vi "Sort_radius.vi"(2 "error in":errorcluster, 3 "unsorted array":dbl[][](array[numeric])) -> (0 "error out":errorcluster, 1 "Array":dbl[][](array[numeric]))   [LabVIEW 2016]
doc: "To vi sortuje tablice 1d pkt w tablice 2d pkt względem promienia , gdzie każdy wiersz to pkt z tym samym promieniem"
uses:
  <vilib>/express/express arith-compare/Formula/XNode/ExpressFormulaBlockNode.xnode
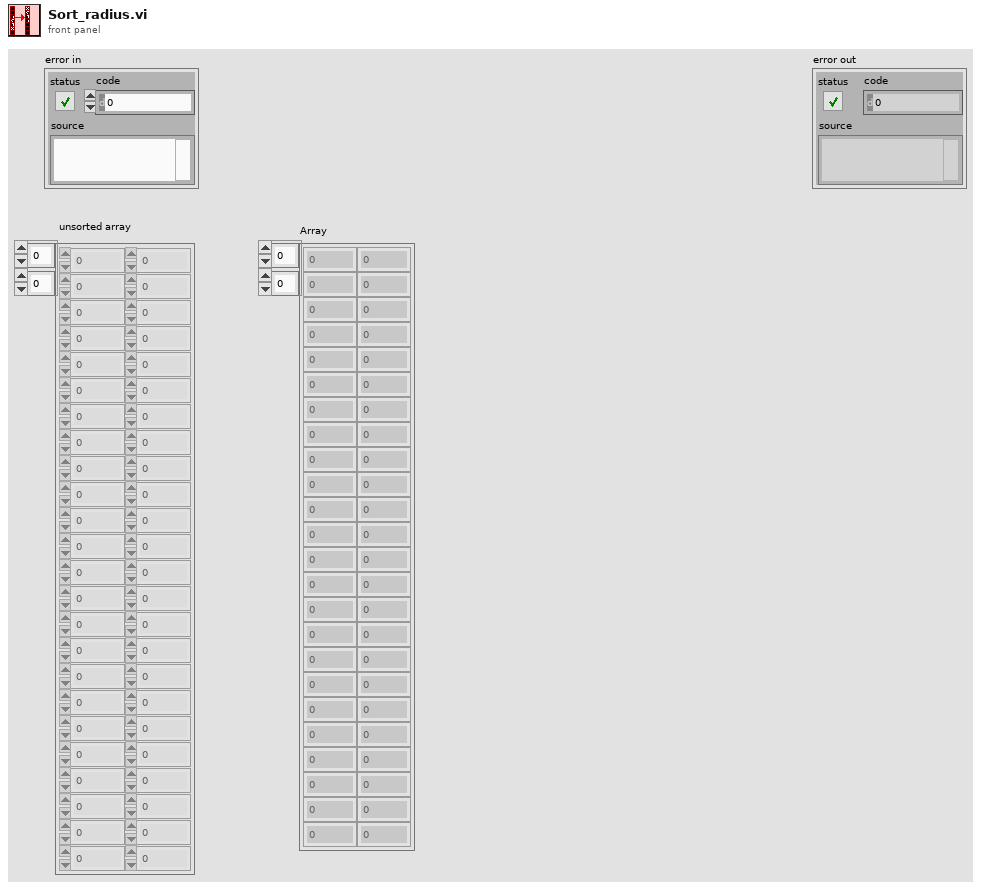
[diagram p1: front panel]
types:
  T1 = cluster{"Result":dbl, "Numeric":dbl, "Numeric":dbl}
  T2 = cluster{"Result":dbl, "Numeric":dbl, "Numeric":dbl}[]
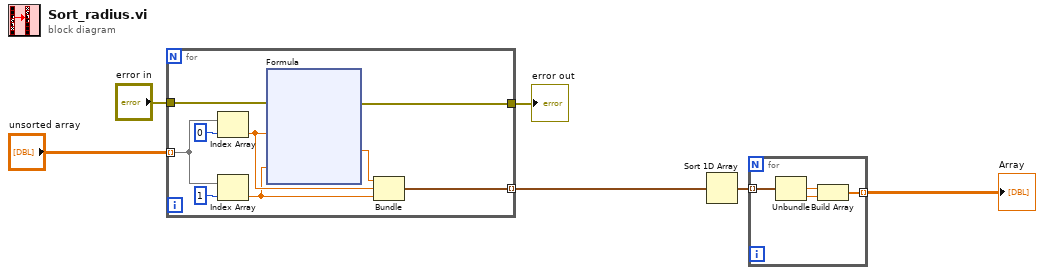
[diagram p0: block diagram]
diagram:
  n1 = for {
    tunnel: "unsorted array" -> [w12] mode=indexing
    tunnel: [w13] -> w4 mode=indexing
    tunnel: "error in" -> [w11]
    tunnel: [w10] -> w5
    n2 = Index Array(array=w12, index=0) -> (element=w9:dbl)
    n3 = Index Array(array=w12, index=1) -> (element=w8:dbl)
    n4 = xnode "Formula"("x"=w9, "y"=w8, "error in (no error)"=w11) -> ("Result"=w7:dbl, "error out"=w10:errorcluster)
    n5 = Bundle("Result"=w7, "Numeric"=w9, "Numeric"=w8) -> (w13:T1)  [unwired: 1 in]
  }
  "error out" <- w5
  n6 = Sort 1D Array(array=w4) -> (sorted array=w3:T2)
  n7 = for {
    tunnel: [w27] -> w1 mode=indexing
    tunnel: w3 -> [w26] mode=indexing
    n8 = Unbundle(w26) -> ("Numeric"=w29:dbl, "Numeric"=w28:dbl)  [unwired: 1 out]
    n9 = Build Array(w29, w28) -> (w27:dbl[])
  }
  "Array" <- w1
